vi "Limit Testing Time.vi"(6 "limit test config":T1={"pass region"=0, "include UL"=TRUE, "include LL"=TRUE} {"pass region" items=["inside limits", "outside limits"]}, 7 "output t0":u32(ring) items=["t0 = limit x0", "t0 = signal in t0"], 8 "error in (no error)":errorcluster, 9 "lower limit":cluster{"x0":dbl, "dx":dbl, "Y":dbl[]}={"x0"=0.0, "dx"=1.0, "Y"=[]} {"Y" format="%.2p"; "dx" format="%.2p"; "x0" format="%.2p"}, 10 "upper limit":cluster{"x0":dbl, "dx":dbl, "Y":dbl[]}={"x0"=0.0, "dx"=1.0, "Y"=[]} {"Y" format="%.2p"; "dx" format="%.2p"; "x0" format="%.2p"}, 11 "signal in":waveform(dbl)) -> (0 "error out":errorcluster, 1 "output values":waveform(dbl)[](array[waveform]), 2 "test results":bool[](array[boolean]), 3 "test passed?":bool, 4 "clearance":T2 {"min clearance" format="%.2p"; "clearance LL" format="%.2p"; "clearance UL" format="%.2p"}, 5 "failures":cluster{"x values":dbl[], "y values":dbl[]} {"y values" format="%.2p"; "x values" format="%.2p"})   [LabVIEW 2020, in "NI_MAPro.lvlib"]
doc: "Performs limit testing on waveform or cluster input data. The VI compares <B>signal in</B> with <B>upper limit</B> and <B>lower limit</B> and ignores any limit input that is not wired. You can wire <B>output values</B> to a graph to view the limits, signal, and failures. Wire data to the <B>signal in</B> input to determine the polymorphic instance to use or manually select the instance."
uses:
  NI_MAPro.lvlib
  NI_MABase.lvlib
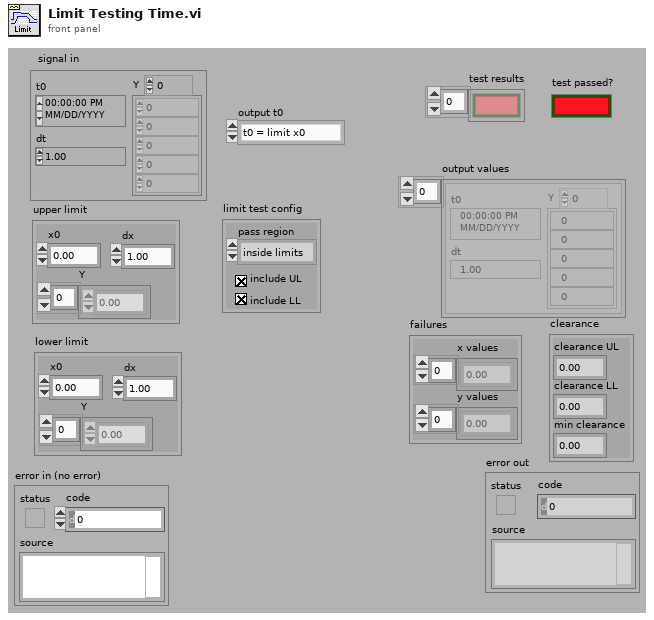
[diagram p1: front panel]
types:
  T1 = cluster{"pass region":i32, "include UL":bool, "include LL":bool}
  T2 = cluster{"clearance UL":dbl, "clearance LL":dbl, "min clearance":dbl}
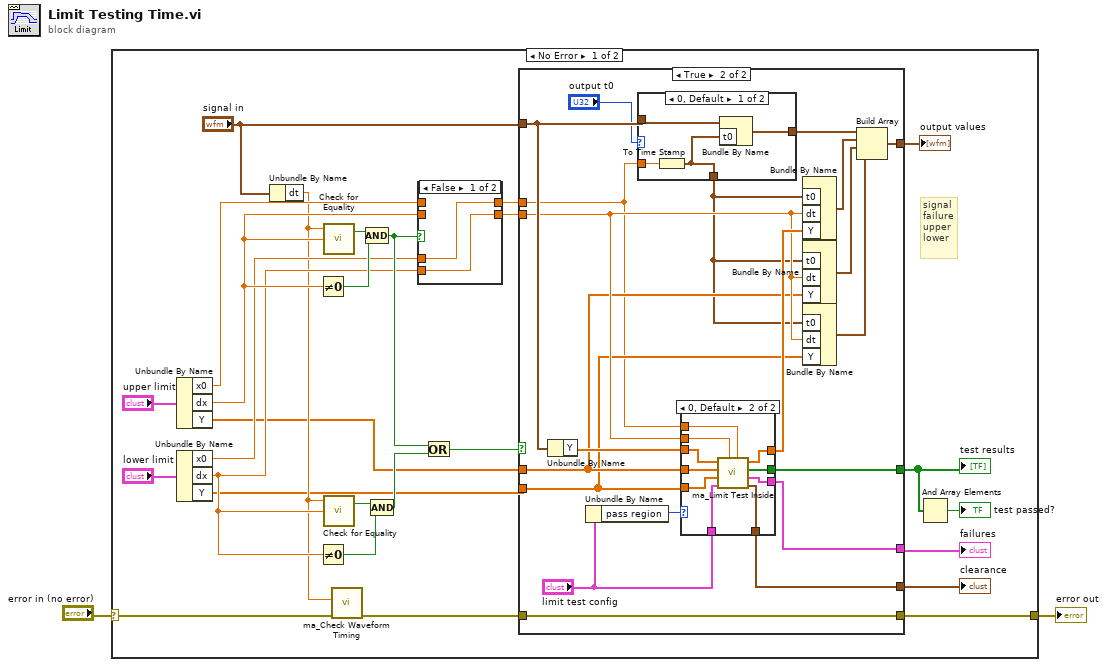
[diagram p0: block diagram]
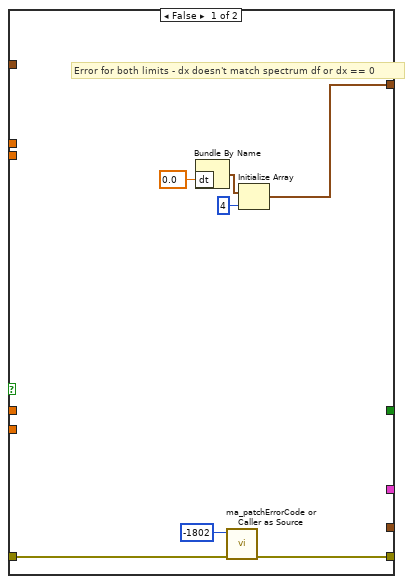
[diagram p3: hidden frame]
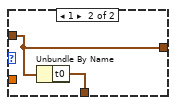
[diagram p4: hidden frame]
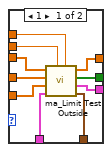
[diagram p5: hidden frame]
diagram:
  n1 = case shown="No Error" "error in (no error)" {
    selector: "error in (no error)" -> [w10 w87]
    tunnel: [w11 w87] -> w1
    frame No Error {
      # "signal\nfailure\nupper\nlower"
      n2 = Unbundle By Name("upper limit") -> ("x0"=w22:dbl, "dx"=w21:dbl, "Y"=w4:dbl[])
      n3 = Unbundle By Name("lower limit") -> ("x0"=w19:dbl, "dx"=w8:dbl, "Y"=w3:dbl[])
      n4 = Unbundle By Name("signal in") -> ("dt"=w5:dbl)
      n5 = Not Equal To 0?(x=w21) -> (x != 0?=w29:bool)
      n6 = Not Equal To 0?(x=w8) -> (x != 0?=w28:bool)
      n7 = call "Check for Equality.vi"("n2"=w21, "n1"=w5) -> ("equal?"=w6:bool)  [unwired: 1 in, 1 out]
      n8 = call "Check for Equality.vi"("n2"=w8, "n1"=w5) -> ("equal?"=w7:bool)  [unwired: 1 in, 1 out]
      n9 = call "ma_Check Waveform Timing.vi"("error in (no error)"=w10, "dt"=w5) -> ("error out"=w9:errorcluster)  [unwired: 1 in, 8 out]
      n10 = Compound Arithmetic op=AND(w6, w29) -> (w20:bool)
      n11 = Compound Arithmetic op=AND(w7, w28) -> (w23:bool)
      n12 = case shown="False" w20 {
        tunnel: w22 -> [_ w33]
        tunnel: w21 -> [_ w32]
        tunnel: w19 -> [w31 _]
        tunnel: w8 -> [w30 _]
        tunnel: [w31 w33] -> w18
        tunnel: [w30 w32] -> w17
        frame False {
        }
        frame True {
        }
      }
      n13 = Or(x=w20, y=w23) -> (x .or. y?=w24:bool)
      n14 = case shown="True" w24 {
        tunnel: [_ w60] -> w15
        tunnel: "signal in" -> [_ w54]
        tunnel: w18 -> [_ w41]
        tunnel: w17 -> [_ w46]
        tunnel: w9 -> [w38 w55]
        tunnel: [w37 w55] -> w11
        tunnel: [w36 w51] -> w16
        tunnel: [_ w59] -> w13
        tunnel: [_ w58] -> w12
        tunnel: w4 -> [_ w45]
        tunnel: w3 -> [_ w44]
        frame False {
          # "Error for both limits - dx doesn't match spectrum df or dx == 0"
          n15 = Bundle By Name("dt"=0.0) -> (w34:waveform(dbl))  [unwired: 1 out]
          n16 = call "ma_patchErrorCode or Caller as Source.vi"("error in (no error)"=w38, "error code"=-1802 ("Error Code")) -> ("error out"=w37:errorcluster)  [unwired: 2 in, 7 out]
          n17 = Initialize Array(w34, 4 ("dimension size")) -> (w36:waveform(dbl)[])
        }
        frame True {
          n18 = Unbundle By Name(w54) -> ("Y"=w53:dbl[])
          n19 = Unbundle By Name("limit test config") -> ("pass region"=w56:i32)
          n20 = case shown="0, Default" "output t0" {
            tunnel: w54 -> [w64 w65]
            tunnel: [w63 w65] -> w50
            tunnel: [w61 w66] -> w42
            tunnel: w41 -> [w62 _]
            frame 0, Default {
              n21 = To Time Stamp(1:w62) -> (0:w61:timestamp)
              n22 = Bundle By Name(cluster=w64, "t0"=w61) -> (w63:waveform(dbl))
            }
            frame 1 {
              n23 = Unbundle By Name(w65) -> ("t0"=w66:timestamp)
            }
          }
          n24 = case shown="0, Default" w56 {
            tunnel: [w76 w80] -> w60
            tunnel: w45 -> [w75 w86]
            tunnel: w44 -> [w74 w85]
            tunnel: [w73 w84] -> w52
            tunnel: [w72 w83] -> w59
            tunnel: [w71 w82] -> w58
            tunnel: "limit test config" -> [w70 w81]
            tunnel: w41 -> [w69 w79]
            tunnel: w46 -> [w68 w78]
            tunnel: w53 -> [w67 w77]
            frame 1 {
              n25 = call "ma_Limit Test Outside.vi"("x0"=w69, "dx"=w68, "limit test config"=w70, "lower"=w74, "upper"=w75, "signal"=w67) -> ("clearance"=w71:T2, "failures"=w72:cluster{"x values":dbl[], "y values":dbl[]}, "test results"=w76:bool[], "Y"=w73:dbl[])  [unwired: 2 out]
            }
            frame 0, Default {
              n26 = call "ma_Limit Test Inside.vi"("x0"=w79, "dx"=w78, "limit test config"=w81, "lower"=w85, "upper"=w86, "signal"=w77) -> ("clearance"=w82:T2, "failures"=w83:cluster{"x values":dbl[], "y values":dbl[]}, "test results"=w80:bool[], "Y"=w84:dbl[])  [unwired: 2 out]
            }
          }
          n27 = Bundle By Name("t0"=w42, "dt"=w46, "Y"=w52) -> (w49:waveform(dbl))  [unwired: 1 out]
          n28 = Bundle By Name("t0"=w42, "dt"=w46, "Y"=w45) -> (w48:waveform(dbl))  [unwired: 1 out]
          n29 = Bundle By Name("t0"=w42, "dt"=w46, "Y"=w44) -> (w47:waveform(dbl))  [unwired: 1 out]
          n30 = Build Array(w50, w49, w48, w47) -> (w51:waveform(dbl)[])
        }
      }
      "output values" <- w16
      "test results" <- w15
      "failures" <- w13
      "clearance" <- w12
      n31 = And Array Elements(Boolean array=w15) -> (logical AND=→"test passed?":bool)
    }
    frame Error {
    }
  }
  "error out" <- w1
